vi "AI_InstantRead.vi"(0 "Task ID":u32, 1 "error in (no error)":errorcluster) -> (2 "Task ID":u32, 3 "Dynamic Data Type":dynamicdata(waveform), 4 "error out":errorcluster)   [LabVIEW 2015]
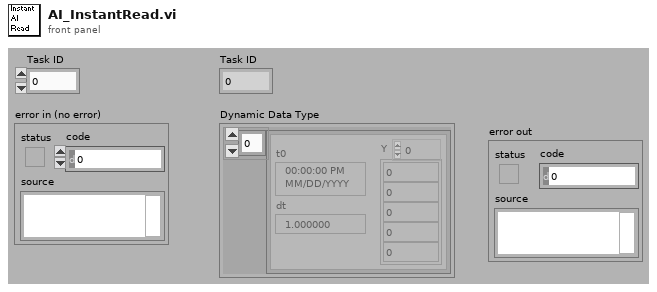
[diagram p1: front panel]
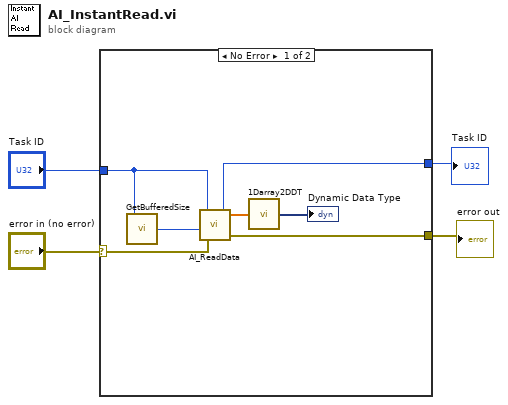
[diagram p0: block diagram]
diagram:
  n1 = case shown="No Error" "error in (no error)" {
    selector: "error in (no error)" -> [w11 w12]
    tunnel: "Task ID" -> [w5 w13]
    tunnel: [w10 w12] -> w3
    tunnel: [w9 w13] -> w2
    frame No Error {
      n2 = call "GetBufferedSize.vi"("Task ID"=w5) -> ("return type"=w6:i32)
      n3 = call "AI_ReadData.vi"("error IO"=w11, "count"=w6, "Task ID"=w5) -> ("error out"=w10:errorcluster, "data"=w8:dbl[], "Task ID"=w9:u32)  [unwired: 1 in]
      n4 = call "1Darray2DDT.vi"("Array"=w8) -> ("Dynamic Data Type"=→"Dynamic Data Type":dynamicdata)
    }
    frame Error {
    }
  }
  "error out" <- w3
  "Task ID" <- w2
